vi "I2C Message Buffer - Create.vi"(8 "error in (no error)":errorcluster) -> (0 "error out":errorcluster)   [LabVIEW 2025, in "I2C Bus Monitor.lvclass"]
uses:
  I2C Bus Monitor.lvclass
  I2C Bus Monitor.lvclass/I2C Bus Monitor.ctl
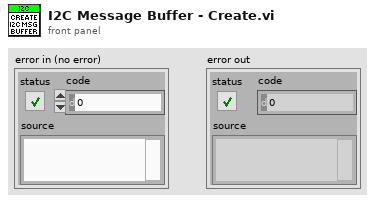
[diagram p1: front panel]
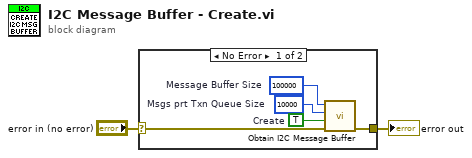
[diagram p0: block diagram]
diagram:
  n1 = case shown="No Error" "error in (no error)" {
    selector: "error in (no error)" -> [w7 w8]
    tunnel: [w6 w8] -> w1
    frame No Error {
      w3 = 100000  # Message Buffer Size
      w4 = 10000  # Msgs prt Txn Queue Size
      w5 = TRUE  # Create
      n2 = call "Obtain I2C Message Buffer.vi"("error in (no error)"=w7, "Create (F)"=w5, "Msgs per Txn Queue Size (10k)"=w4, "Message Buffer Size (100k)"=w3) -> ("error out"=w6:errorcluster)  [unwired: 5 in, 2 out]
    }
    frame Error {
    }
  }
  "error out" <- w1
